vi "SQLite Add Saving Test.vi"(7 "Test DB Set Up Command":string, 8 "Error In (no error)":errorcluster, 11 "SQLite DB Operator In":refnum<class "SQLite DB Operator.lvclass">) -> (0 "Error Out":errorcluster, 3 "SQLite DB Operator Out":refnum<class "SQLite DB Operator.lvclass">)   [LabVIEW 2023]
uses:
  Clasess/SQLite DB Operator/SQLite DB Operator.lvclass
  Clasess/DB Records/Expenses Tracker Saving/Public/Ctrls/Saving.ctl
  Clasess/DB Records/Expenses Tracker Saving/Expenses Tracker Saving.lvclass
  H:/Desktop/LabVIEW/LabView Repo/Expenses-Tracker-DB-Operator/Interfaces/Expenses Tracker Record/Expenses Tracker Record.lvclass
  <vilib>/drjdpowell/SQLite Library/SQL Connection/Execute SQL (1D Cluster).vi
  <vilib>/addons/_JKI Toolkits/Caraya/classes/Test/Test.lvclass
  <vilib>/drjdpowell/SQLite Library/SQLite.lvlib
  H:/Desktop/LabVIEW/LabView Repo/Expenses-Tracker-DB-Operator/Clasess/DB Records/Expenses Tracker Saving/Expenses Tracker Saving.lvclass
  <vilib>/drjdpowell/SQLite Library/SQL Connection/Connection.lvclass
  Support/Adding/Add Record Assert Error.vi
  Support/Adding/Add Record Assert Not Error.vi
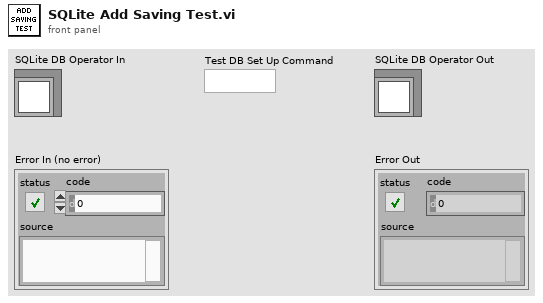
[diagram p1: front panel]
types:
  T1 = typedef "Expenses Tracker Saving.lvclass/Saving.ctl" = cluster{"ID":u32, "Saving_goal":u32, "Value":dbl, "Date_of_entry":timestamp, "Description":string}
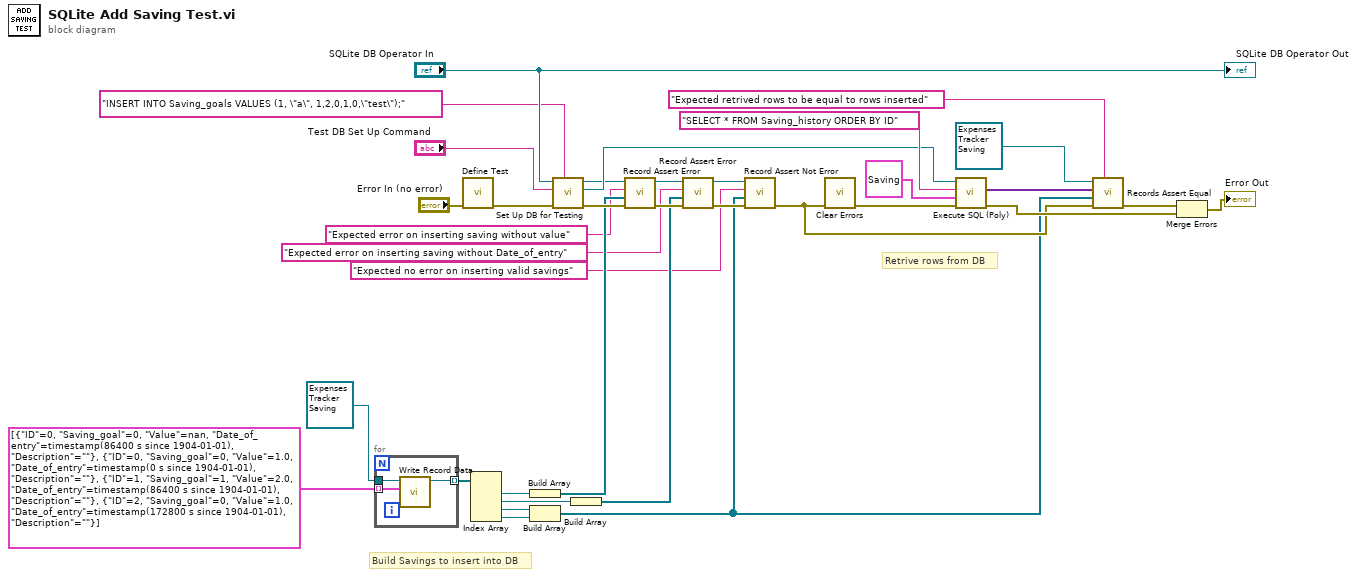
[diagram p0: block diagram]
diagram:
  # "Retrive rows from DB"
  # "Build Savings to insert into DB"
  n1 = for {
    tunnel: T1[] [{"ID"=0, "Saving_goal"=0, "Value"=nan, "Date_of_entry"=timestamp(86400 s since 1904-01-01), "Description"=""}, {"ID"=0, "Saving_goal"=0, "Value"=1.0, "Date_of_entry"=timestamp(0 s since 1904-01-01), "Description"=""}, {"ID"=1, "Saving_goal"=1, "Value"=2.0, "Date_of_entry"=timestamp(86400 s since 1904-01-01), "Description"=""}, {"ID"=2, "Saving_goal"=0, "Value"=1.0, "Date_of_entry"=timestamp(172800 s since 1904-01-01), "Description"=""}] ("Array") -> [w38] mode=indexing
    tunnel: refnum<class "Expenses Tracker Saving.lvclass"> refnum ("Expenses Tracker Category") -> [w36]
    tunnel: [w37] -> w33 mode=indexing
    n2 = call-dynamic "Write Record Data.vi"("Record"=w38, "Expenses Tracker Saving In"=w36) -> ("Expenses Tracker Saving Out"=w37:refnum<class "Expenses Tracker Saving.lvclass">)  [unwired: 8 in, 1 out]
  }
  n3 = call <vilib>:"Define Test.vi"("error in (no error)"="Error In (no error)") -> ("error out"=w26:errorcluster)  [unwired: 9 in, 1 out]
  n4 = Index Array(array=w33) -> (element #1=w14:refnum<class "Expenses Tracker Saving.lvclass">, element #2=w10:refnum<class "Expenses Tracker Saving.lvclass">, element #3=w7:refnum<class "Expenses Tracker Saving.lvclass">, element #4=w2:refnum<class "Expenses Tracker Saving.lvclass">)  [unwired: 4 in]
  n5 = Build Array(w14) -> (w13:refnum<class "Expenses Tracker Saving.lvclass">[])
  n6 = Build Array(w7, w2) -> (w1:refnum<class "Expenses Tracker Saving.lvclass">[])
  n7 = call "Set Up DB for Testing.vi"("Additional Set Up Commands"="INSERT INTO Saving_goals VALUES (1, \"a\", 1,2,0,1,0,\"test\");", "Error In (no error)"=w26, "Test DB Set Up Command"="Test DB Set Up Command", "SQLite DB Operator In"="SQLite DB Operator In") -> ("Error Out"=w16:errorcluster, "SQLite Connection"=w30:refnum<class "Connection.lvclass">, "SQLite DB Operator Out"=w12:refnum<class "SQLite DB Operator.lvclass">)  [unwired: 5 in]
  n8 = Build Array(w10) -> (w9:refnum<class "Expenses Tracker Saving.lvclass">[])
  n9 = call-poly "Record Assert Error.vi"("Error In"=w16, "Records"=w13, "Assertion Label"="Expected error on inserting saving without value" ("Label (VI Title)"), "SQLite DB Operator In"=w12) -> ("Error Out"=w19:errorcluster, "SQLite DB Operator Out"=w20:refnum<class "SQLite DB Operator.lvclass">)  [unwired: 6 in]
  n10 = call-poly "Record Assert Error.vi"("Error In"=w19, "Records"=w9, "Assertion Label"="Expected error on inserting saving without Date_of_entry" ("Label (VI Title)"), "SQLite DB Operator In"=w20) -> ("Error Out"=w17:errorcluster, "SQLite DB Operator Out"=w18:refnum<class "SQLite DB Operator.lvclass">)  [unwired: 6 in]
  n11 = call-poly "Record Assert Not Error.vi"("Error In"=w17, "Records"=w1, "Assertion Label"="Expected no error on inserting valid savings" ("Label (VI Title)"), "SQLite DB Operator In"=w18) -> ("Error Out"=w15:errorcluster)  [unwired: 6 in, 1 out]
  n12 = call <vilib>:"Clear Errors.vi"("error in (no error)"=w15) -> ("error out"=w21:errorcluster)  [unwired: 5 in, 1 out]
  n13 = call-poly <vilib>:"Execute SQL (Poly).vi"("error in (no error)"=w21, "Cluster (or Array of Clusters)"=T1 {"ID"=0, "Saving_goal"=0, "Value"=0.0, "Date_of_entry"=timestamp(0 s since 1904-01-01), "Description"=""} ("Saving"), "SQL"="SELECT * FROM Saving_history ORDER BY ID", "SQLite Connection in"=w30) -> ("error out"=w22:errorcluster, "Result Set (Array of Clusters)"=w6:variant[])  [unwired: 5 in, 1 out]
  n14 = call "Records Assert Equal.vi"("Assertion Label"="Expected retrived rows to be equal to rows inserted" ("Label (VI Title)"), "Error In"=w15, "Correct Records"=w1, "Typedef Records"=w6, "Expenses Tracker Record In"=refnum<class "Expenses Tracker Saving.lvclass"> refnum ("Expenses Tracker Category")) -> ("Error Out"=w23:errorcluster)  [unwired: 6 in]
  n15 = Merge Errors(w23, w22) -> (→"Error Out":errorcluster)
  "SQLite DB Operator Out" <- "SQLite DB Operator In"
